vi "Read configuration.vi"(7 "force loading?":bool=TRUE, 8 "error in (no error)":errorcluster, 11 "Autofocus in":refnum<class "Autofocus.lvclass">) -> (0 "error out":errorcluster, 3 "Autofocus out":refnum<class "Autofocus.lvclass">)   [LabVIEW 2012, in "Autofocus.lvclass"]
doc: "Reads the XML-based configuration file and populates the configuration cluster accordingly. Configuration file name is <component ID>.xml."
uses:
  Autofocus.lvclass
  <vilib>/Distrio/Murmex/Murmex/Murmex.lvclass
  Autofocus.lvclass/Autofocus.ctl
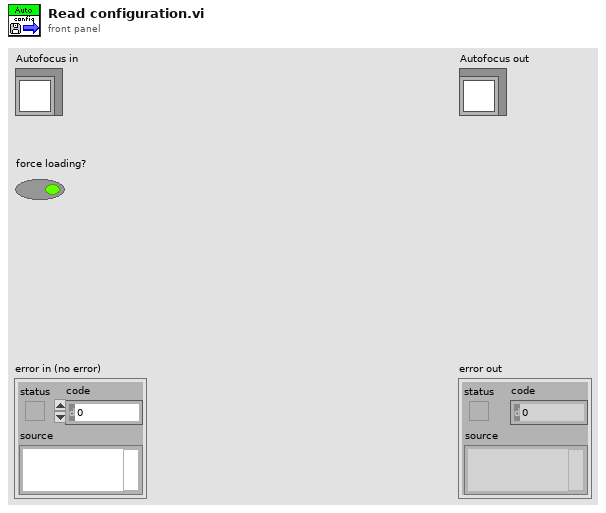
[diagram p1: front panel]
types:
  T1 = typedef "Autofocus.lvclass/configuration cluster.ctl" = cluster{"Camera component name":string, "Stages component name":string, "Tomo component name":string, "Epsilon (HC)":dbl, "Epsilon (GS)":dbl, "Number of subregions":T2}
  T2 = typedef "Autofocus.lvclass/number of subregions.ctl" = i32
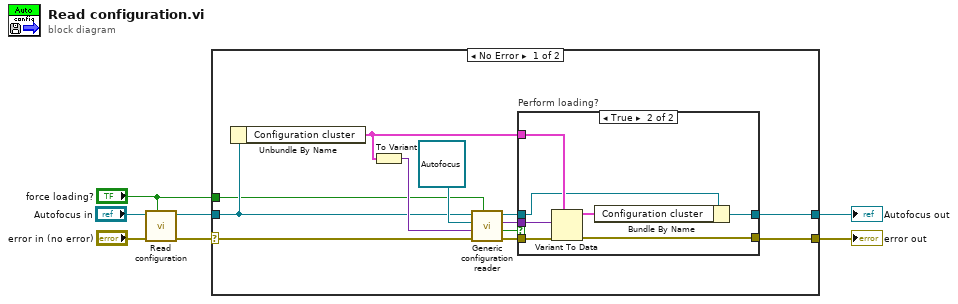
[diagram p0: block diagram]
diagram:
  n1 = call-parent "Read configuration.vi"("force loading?"="force loading?", "error in (no error)"="error in (no error)", "Murmex in"="Autofocus in") -> ("error out"=w5:errorcluster, "Murmex out"=w4:refnum<class "Autofocus.lvclass">)  [unwired: 7 in]
  n2 = case shown="No Error" w5 {
    selector: w5 -> [w17 w30]
    tunnel: w4 -> [w16 w29]
    tunnel: "force loading?" -> [w15 _]
    tunnel: [w13 w30] -> w2
    tunnel: [w8 w29] -> w1
    frame No Error {
      n3 = Unbundle By Name(w16) -> ("Configuration cluster"=w12:T1)
      n4 = To Variant(anything=w12) -> (Variant=w18:variant)
      n5 = call <vilib>:"Generic configuration reader.vi"("force loading?"=w15, "error in (no error)"=w17, "configuration cluster variant"=w18, "inheritance level"=refnum<class "Autofocus.lvclass"> refnum ("Autofocus.lvclass"), "Murmex in"=w16) -> ("error out"=w14:errorcluster, "loaded?"=w9:bool, "configuration data (variant)"=w10:variant, "Murmex out"=w11:refnum<class "Autofocus.lvclass">)  [unwired: 3 in]
      n6 = case "Perform loading?" shown="True" w9 {
        tunnel: w12 -> [_ w28]
        tunnel: [w21 w26] -> w13
        tunnel: [w20 w25] -> w8
        tunnel: w14 -> [w21 w22]
        tunnel: w11 -> [w20 w24]
        tunnel: w10 -> [_ w23]
        frame False {
        }
        frame True {
          n7 = Variant To Data(error in=w22, type=w28, Variant=w23) -> (data=w27:T1, error out=w26:errorcluster)
          n8 = Bundle By Name(cluster=w24, "Configuration cluster"=w27) -> (w25:refnum<class "Autofocus.lvclass">)
        }
      }
    }
    frame Error {
    }
  }
  "error out" <- w2
  "Autofocus out" <- w1
